vi "create tomo file name.vi"(8 "error in (no error)":errorcluster, 10 "filename":string, 11 "Autofocus in":refnum<class "Autofocus.lvclass">) -> (0 "error out":errorcluster, 2 "tomo path":path, 3 "Autofocus out":refnum<class "Autofocus.lvclass">)   [LabVIEW 2012, in "Autofocus.lvclass"]
uses:
  Autofocus.lvclass
  Autofocus.lvclass/Autofocus.ctl
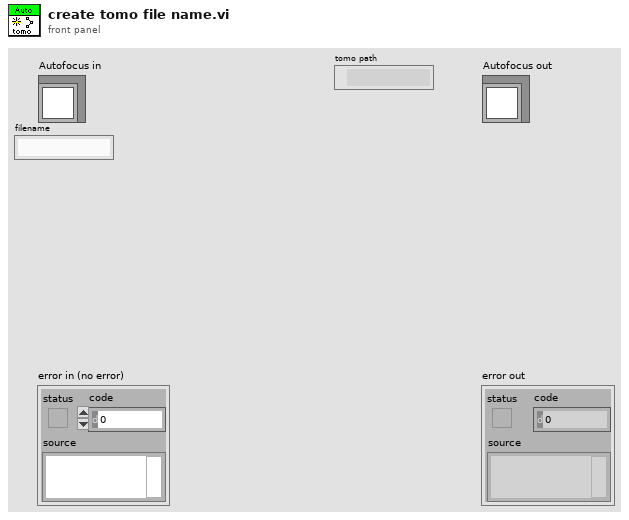
[diagram p1: front panel]
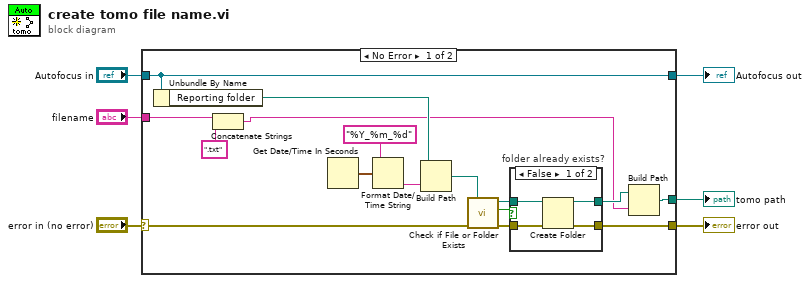
[diagram p0: block diagram]
diagram:
  n1 = case shown="No Error" "error in (no error)" {
    selector: "error in (no error)" -> [w16 w30]
    tunnel: [w12 w30] -> w5
    tunnel: [w22 w29] -> w3
    tunnel: "Autofocus in" -> [w22 w29]
    tunnel: [w11 _] -> w2
    tunnel: "filename" -> [w8 _]
    frame No Error {
      n2 = Unbundle By Name(w22) -> ("Reporting folder"=w19:path)
      n3 = Concatenate Strings(w8, ".txt" ("string")) -> (w7:string)
      n4 = Get Date/Time In Seconds() -> (seconds since 1Jan1904=w21:timestamp)
      n5 = Format Date/Time String(time format string (%c)="%Y_%m_%d", seconds (now)=w21) -> (date/time string=w18:string)  [unwired: 1 in]
      n6 = Build Path(base path=w19, name or relative path=w18) -> (appended path=w17:path)
      n7 = call <vilib>:"Check if File or Folder Exists.vi"("error in (no error)"=w16, "path"=w17) -> ("error out"=w15:errorcluster, "file or folder exists?"=w13:bool, "dup path"=w14:path)  [unwired: 7 in]
      n8 = case "folder already exists?" shown="False" w13 {
        tunnel: [w24 w28] -> w12
        tunnel: w15 -> [w26 w28]
        tunnel: w14 -> [w25 w27]
        tunnel: [w23 w27] -> w10
        frame False {
          n9 = Create Folder(path (use dialog)=w25, error in=w26) -> (created path=w23:path, error out=w24:errorcluster)  [unwired: 1 in, 1 out]
        }
        frame True {
        }
      }
      n10 = Build Path(base path=w10, name or relative path=w7) -> (appended path=w11:path)
    }
    frame Error {
    }
  }
  "error out" <- w5
  "Autofocus out" <- w3
  "tomo path" <- w2
